vi "load_name.vi"(8 "error in (no error)":errorcluster, 11 "toml":string) -> (0 "error out":errorcluster, 2 "remaining string":string, 3 "name":string[](array[string]))   [LabVIEW 2017, in "rpacini_toml.lvlib"]
uses:
  rpacini_toml.lvlib
  <vilib>/regexp/Match Regular Expression.xnode
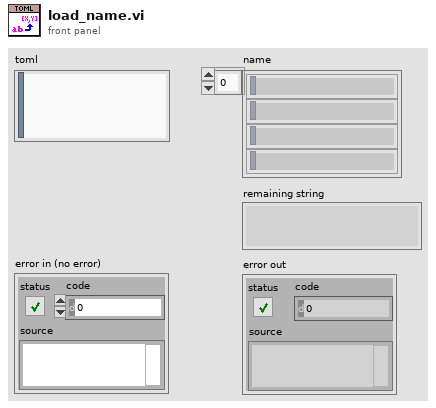
[diagram p1: front panel]
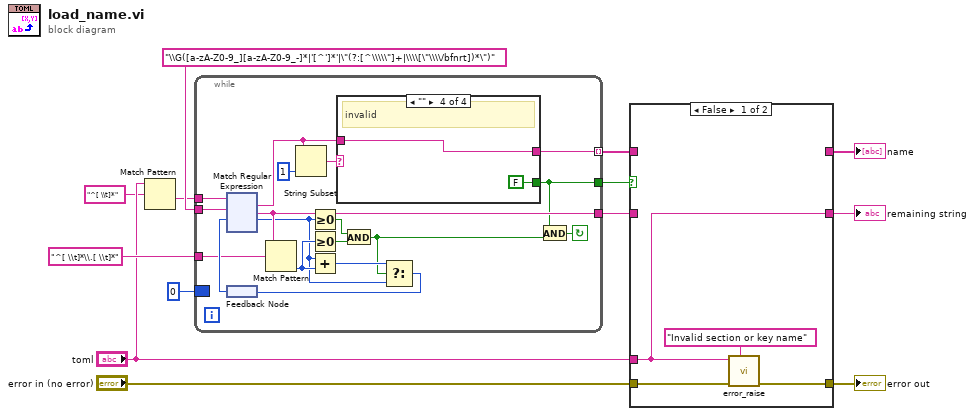
[diagram p0: block diagram]
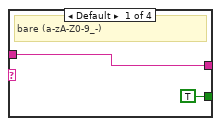
[diagram p3: hidden frame]
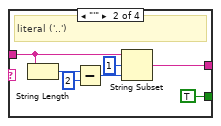
[diagram p4: hidden frame]
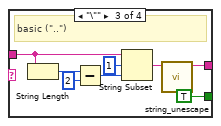
[diagram p5: hidden frame]
diagram:
  n1 = Match Pattern(string="toml", regular expression="^[ \\t]*") -> (after substring=w2:string)  [unwired: 1 in, 3 out]
  n2 = while {
    tunnel: w2 -> [w28]
    tunnel: "\\G([a-zA-Z0-9_][a-zA-Z0-9_-]*|'[^']*'|\"(?:[^\\\\\"]+|\\\\[\"\\\\/bfnrt])*\")" ("regular expression") -> [w31]
    border: 0 ("offset (0)") -> [_]
    tunnel: [w27] -> w4
    tunnel: [w19] -> w6 mode=indexing
    tunnel: "^[ \\t]*\\.[ \\t]*" ("regular expression") -> [w26]
    tunnel: [w14] -> w8
    stop <- w15 continue-if-true
    n3 = feedback #1() -> (w29:i32)
    n4 = xnode "Match Regular Expression"("input string"=w28, "regular expression"=w31, "offset (0)"=w29) -> ("whole match"=w18:string, "after match"=w27:string, "offset past match"=w17:i32)  [unwired: 3 in, 2 out]
    n5 = Match Pattern(string=w27, regular expression=w26) -> (offset past match=w25:i32)  [unwired: 1 in, 3 out]
    n6 = String Subset(string=w18, length (rest)=1 ("length (rest)")) -> (substring=w20:string)  [unwired: 1 in]
    n7 = Greater Or Equal To 0?(x=w17) -> (x >= 0?=w30:bool)
    n8 = Greater Or Equal To 0?(x=w25) -> (x >= 0?=w23:bool)
    n9 = Add(x=w17, y=w25) -> (x+y=w24:i32)
    n10 = case shown="\"\"" w20 {
      tunnel: [w33 w40 w42 w50] -> w19
      tunnel: w18 -> [w33 w38 w47 w50]
      tunnel: [TRUE TRUE TRUE FALSE] -> w14
      frame Default {
        # "bare (a-zA-Z0-9_-)"
      }
      frame "'" {
        # "literal ('..')"
        n11 = String Length(string=w38) -> (length=w37:i32)
        n12 = Subtract(x=w37, y=2 ("x")) -> (x-y=w36:i32)
        n13 = String Subset(string=w38, offset (0)=1, length (rest)=w36) -> (substring=w40:string)
      }
      frame "\"" {
        # "basic (\"..\")"
        n14 = String Length(string=w47) -> (length=w46:i32)
        n15 = Subtract(x=w46, y=2 ("x")) -> (x-y=w45:i32)
        n16 = String Subset(string=w47, offset (0)=1, length (rest)=w45) -> (substring=w43:string)
        n17 = call "string_unescape.vi"("escaped string"=w43) -> ("string out"=w42:string)  [unwired: 9 in, 1 out]
      }
      frame "" {
        # "invalid"
      }
    }
    n18 = And(x=w30, y=w23) -> (x .and. y?=w16:bool)
    n19 = Select(t=w24, s=w16, f=w17) -> (s? t:f=w22:i32)
    n20 = feedback-in #1(w22) -> ()
    n21 = And(x=w14, y=w16) -> (x .and. y?=w15:bool)
  }
  n22 = case shown="False" w8 {
    tunnel: "error in (no error)" -> [w168 w169]
    tunnel: [w167 w169] -> w9
    tunnel: [_ w171] -> w7
    tunnel: w6 -> [_ w171]
    tunnel: [w165 w170] -> w5
    tunnel: w4 -> [_ w170]
    tunnel: "toml" -> [w165 _]
    frame False {
      n23 = call "error_raise.vi"("message"="Invalid section or key name", "error in (no error)"=w168, "toml"=w165) -> ("error out"=w167:errorcluster)  [unwired: 8 in]
    }
    frame True {
    }
  }
  "error out" <- w9
  "name" <- w7
  "remaining string" <- w5
